vi "Inst.MOTOR.RW.vi"(8 "error in (no error)":errorcluster, 10 "Data in":string, 11 "Inst.MOTOR in":refnum<class "Inst.MOTOR.lvclass">) -> (0 "error out":errorcluster, 2 "read buffer":string, 3 "Inst.MOTOR out":refnum<class "Inst.MOTOR.lvclass">)   [LabVIEW 2019, in "Inst.MOTOR.lvclass"]
uses:
  Inst.MOTOR.lvclass
  Inst.MOTOR.lvclass/Inst.MOTOR.ctl
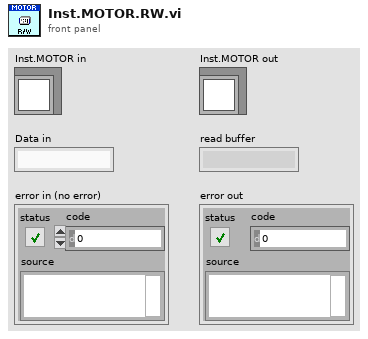
[diagram p1: front panel]
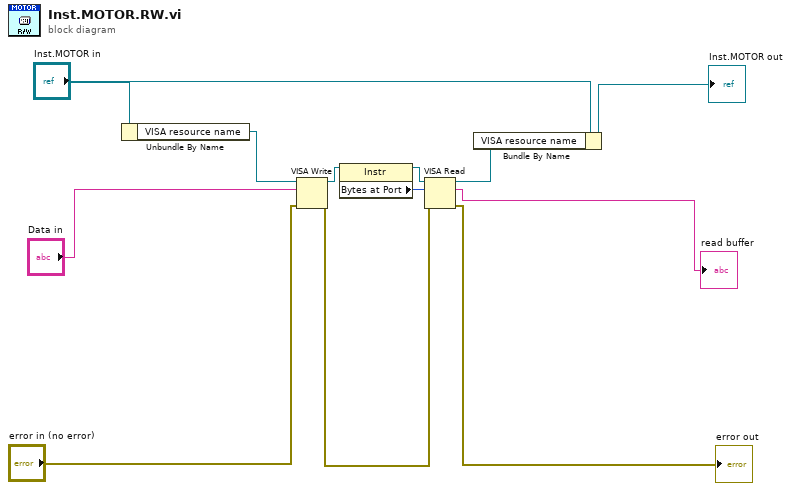
[diagram p0: block diagram]
diagram:
  n1 = Unbundle By Name("Inst.MOTOR in") -> ("VISA resource name"=w5:refnum<visa-resource-name>)
  n2 = VISA Write(VISA resource name=w5, write buffer="Data in", error in (no error)="error in (no error)") -> (VISA resource name out=w2:refnum<visa-resource-name>, error out=w7:errorcluster)  [unwired: 1 out]
  n3 = property class="Instr"(reference=w2) -> (reference out=w1:refnum<visa-resource-name>, "Bytes at Port"=w3:u32)  [unwired: 1 in, 1 out]
  n4 = VISA Read(VISA resource name=w1, byte count=w3, error in (no error)=w7) -> (VISA resource name out=w9:refnum<visa-resource-name>, read buffer=→"read buffer":string, error out=→"error out":errorcluster)  [unwired: 1 out]
  n5 = Bundle By Name(cluster="Inst.MOTOR in", "VISA resource name"=w9) -> (→"Inst.MOTOR out":refnum<class "Inst.MOTOR.lvclass">)
